vi "_Read.vi"(8 "error in":errorcluster, 11 "fd":u64) -> (0 "error out":errorcluster, 2 "MgErr":i32, 3 "buf":string)   [LabVIEW 2020, in "NI_Subprocess.lvlib" / "Subprocess.lvclass"]
doc: "Reads data from the specified file. The read operation is nonblocking."
uses:
  <vilib>/Subprocess/Subprocess/Subprocess.lvclass
  lviosrg.dll
  <vilib>/ErrorRing/Error Ring.xnode
panel:
  out "errno":i32
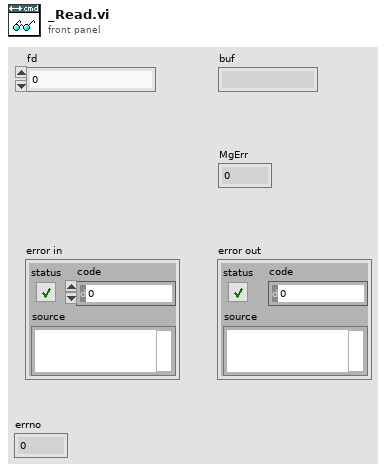
[diagram p1: front panel]
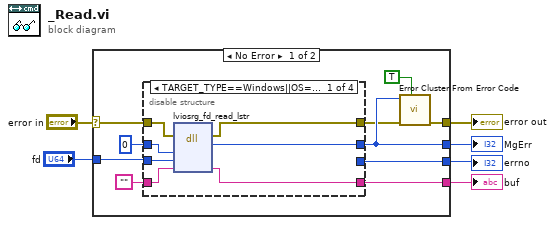
[diagram p0: block diagram]
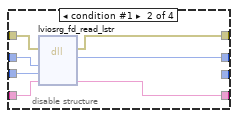
[diagram p2: hidden frame]
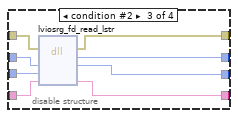
[diagram p3: hidden frame]
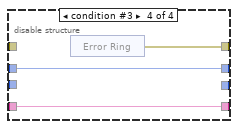
[diagram p4: hidden frame]
diagram:
  n1 = case shown="No Error" "error in" {
    selector: "error in" -> [w12 w46]
    tunnel: [w7 w46] -> w6
    tunnel: [w16 _] -> w5
    tunnel: "fd" -> [w15 _]
    tunnel: [w9 _] -> w3
    tunnel: [w11 _] -> w1
    frame No Error {
      n2 = disable-structure shown="TARGET_TYPE==Windows||OS==Win" {
        disable-tunnel: [w23 w30 w38 w39] -> w8
        disable-tunnel: w12 -> [w22 w29 w37 _]
        disable-tunnel: [w21 w28 w36 w41] -> w16
        disable-tunnel: w15 -> [w20 w27 w35 _]
        disable-tunnel: "" -> [w19 w26 w34 w41]
        disable-tunnel: [w18 w25 w33 w40] -> w9
        disable-tunnel: 0 ("errno") -> [w17 w24 w32 w40]
        disable-tunnel: [_ _ w31 _] -> w11
        frame condition #0 (active) {
          n3 = dll-call lib="lviosrg.*" fn="lviosrg_fd_read_lstr"(error in=w22, "errno"=w17, "read_fd"=w20, "buf"=w19) -> (error out=w23:errorcluster, "return type"=w18:i32, "buf"=w21:string)  [unwired: 4 in, 1 out]
        }
        frame condition #1 {
          n4 = dll-call lib="lviosrg.*" fn="lviosrg_fd_read_lstr"(error in=w29, "errno"=w24, "read_fd"=w27, "buf"=w26) -> (error out=w30:errorcluster, "return type"=w25:i32, "buf"=w28:string)  [unwired: 4 in, 1 out]
        }
        frame condition #2 {
          n5 = dll-call lib="lviosrg.*" fn="lviosrg_fd_read_lstr"(error in=w37, "errno"=w32, "read_fd"=w35, "buf"=w34) -> (error out=w38:errorcluster, "MgErr"=w33:i32, "errno"=w31:i32, "buf"=w36:string)  [unwired: 3 in, 1 out]
        }
        frame condition #3 {
          n6 = xnode "Error Ring"() -> ("error out"=w39:errorcluster)
        }
      }
      n7 = call <vilib>:"Error Cluster From Error Code.vi"("show call chain? (False)"=TRUE, "error in (no error)"=w8, "error code (0)"=w9) -> ("error out"=w7:errorcluster)  [unwired: 6 in]
    }
    frame Error {
    }
  }
  "error out" <- w6
  "buf" <- w5
  "MgErr" <- w3
  "errno" <- w1
